vi "System Init.vi"(8 "error in (no error)":errorcluster) -> (0 "error out":errorcluster)   [LabVIEW 2013]
uses:
  System Status/Status FG Enum.ctl
  Globals/Average Sector Data.vi
  Message Passing/Main MsgQ.lvlib
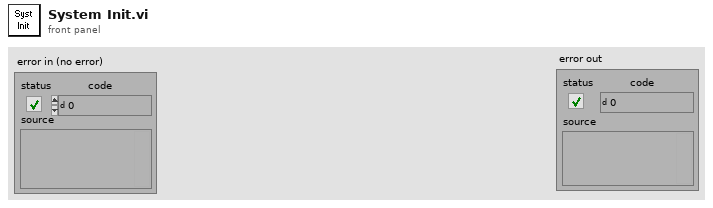
[diagram p1: front panel]
types:
  T1 = enum16{"Config Files", "MSG Queues", "Initialize FG"}[]
  T2 = typedef "Status FG Enum.ctl" = enum16{"Reset", "Read", "Write"}
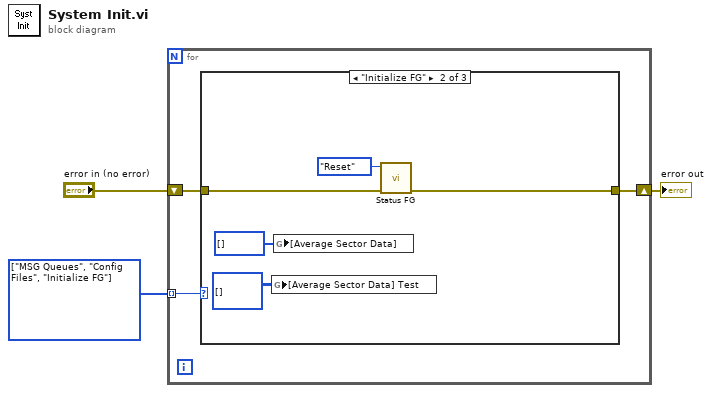
[diagram p0: block diagram]
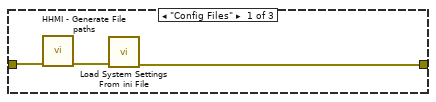
[diagram p2: hidden frame]
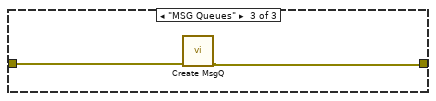
[diagram p3: hidden frame]
diagram:
  w3 = T1 [enum."MSG Queues", enum."Config Files", enum."Initialize FG"] items=["Config Files", "MSG Queues", "Initialize FG"]
  n1 = for {
    tunnel: w3 -> [w6] mode=indexing
    shift-right: [w4] -> w1
    shift-left: "error in (no error)" -> [w5]
    n2 = case shown="\"Initialize FG\"" w6 {
      tunnel: w5 -> [w8 w13 w16]
      tunnel: [w7 w11 w15] -> w4
      frame "Config Files" {
        n3 = call "HHMI - Generate File paths.vi"("error in"=w8) -> ("error out"=w9:errorcluster)  [unwired: 8 in, 2 out]
        n4 = call "Load System Settings From ini File.vi"("error in"=w9) -> ("error out"=w7:errorcluster)  [unwired: 9 in, 1 out]
      }
      frame "Initialize FG" {
        n5 = global write "Average Sector Data.vi" "[Average Sector Data] Test"(u8[][] [] ("[Average Sector Data] Test")) -> ()
        n6 = global write "Average Sector Data.vi" "[Average Sector Data]"(u8[] [] ("[Average Sector Data]")) -> ()
        n7 = call "Status FG.vi"("error in (no error)"=w13, "Operation"=Status_FG_Enum."Reset") -> ("error out"=w11:errorcluster)  [unwired: 8 in, 1 out]
      }
      frame "MSG Queues" {
        n8 = call "Create MsgQ.vi"("error in (no error)"=w16) -> ("error out"=w15:errorcluster)  [unwired: 10 in]
      }
    }
  }
  "error out" <- w1
